vi "MP-285 Set Origin.vi"(2 "error in (no error)":errorcluster, 3 "VISA resource name":refnum<visa-resource-name>) -> (0 "error out":errorcluster, 1 "VISA resource name out":refnum<visa-resource-name>)   [LabVIEW 2010]
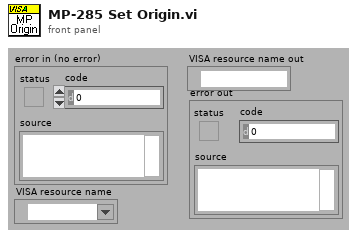
[diagram p1: front panel]
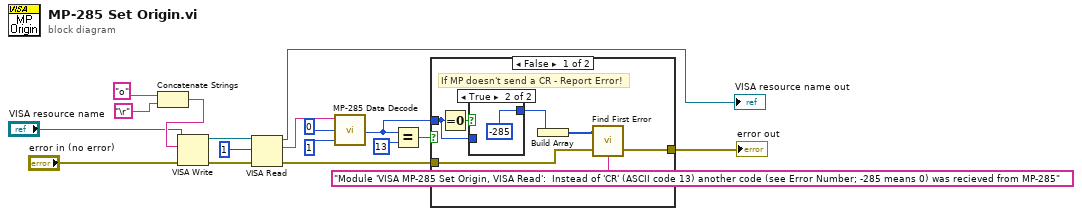
[diagram p0: block diagram]
diagram:
  n1 = Concatenate Strings("o", "\r") -> (w15:string)
  n2 = VISA Write(VISA resource name="VISA resource name", write buffer=w15, error in (no error)="error in (no error)") -> (VISA resource name out=w14:refnum<visa-resource-name>, error out=w13:errorcluster)  [unwired: 1 out]
  n3 = VISA Read(VISA resource name=w14, byte count=1, error in (no error)=w13) -> (VISA resource name out=→"VISA resource name out":refnum<visa-resource-name>, read buffer=w5:string, error out=w8:errorcluster)  [unwired: 1 out]
  n4 = call "MP-285 Data Decode.vi"("Input: lenght"=1, "Input: offset"=0, "Input: Data string"=w5) -> ("Output: Decoded Data"=w9:i32)
  n5 = Equal?(x=w9, y=13) -> (x = y?=w10:bool)
  n6 = case shown="False" w10 {
    tunnel: [w24 w27] -> w3
    tunnel: w9 -> [w20 _]
    tunnel: w8 -> [w18 w27]
    frame False {
      # "If MP doesn't send a CR - Report Error!"
      n7 = Equal To 0?(x=w20) -> (x = 0?=w21:bool)
      n8 = case shown="True" w21 {
        tunnel: w20 -> [w25 _]
        tunnel: [w25 -285] -> w19
        frame False {
        }
        frame True {
        }
      }
      n9 = Build Array(w19) -> (w22:i32[])
      n10 = call <vilib>:"Find First Error.vi"("error in (no error)"=w18, "source messages"="Module 'VISA MP-285 Set Origin, VISA Read':  Instead of 'CR' (ASCII code 13) another code (see Error Number; -285 means 0) was recieved from MP-285", "error codes"=w22) -> ("error out"=w24:errorcluster)  [unwired: 2 out]
    }
    frame True {
      # "TRUE: CR was received - NO Errors"
    }
  }
  "error out" <- w3
